vi "ProdaNG.CheckProductExists.vi"(8 "error in (no error)":errorcluster, 9 "serialNumber":string, 10 "ID":T2, 11 "dbHandle":i32) -> (0 "error out":errorcluster, 1 "ProductID":T1, 2 "Results exist?":bool, 3 "dbHandle out":i32, 5 "Prod exist?":bool, 7 "Prod status":i32)   [LabVIEW 2016]
doc: "This function returns a product structure for a product, which is identified by a part and a serial number.\nImportant information: The field 'individual' was taken over from the field 'allgemein' of the legacy data directly. Because of this most products have the value 0 further on and only a few the value 1. \nParameter:\nhandle is an Integer, which is returned by the function Login() at the creation of a new connection.\nwabcoPartId is the Id of the part.\nserialNumber is the serial number of the product for the part above.\nproduct is a pointer on a product structure, which is filled if the returncode is 0. The structure must be defined in the calling program.\n\nReturncodes:\n0 No error\n< 0 ORACLE Error code\n6 (ERROR_INVALID_HANDLE) in case of an invalid handle\n1403 Record does not exist"
uses:
  Controls/ProdaNG.Identification.ctl
  Controls/ProdaNG.Product.ctl
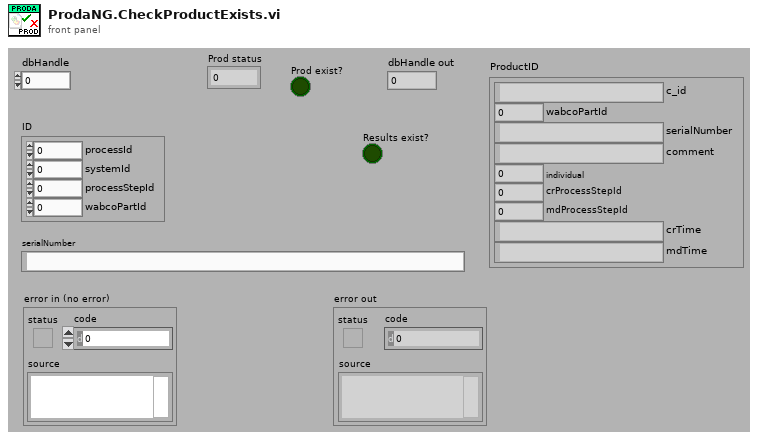
[diagram p1: front panel]
types:
  T1 = typedef "ProdaNG.Product.ctl" = cluster{"c_id":string, "wabcoPartId":i32, "serialNumber":string, "comment":string, "individual":i32, "crProcessStepId":i32, "mdProcessStepId":i32, "crTime":string, "mdTime":string}
  T2 = typedef "ProdaNG.Identification.ctl" = cluster{"processId":i32, "systemId":i32, "processStepId":i32, "wabcoPartId":i32}
  T3 = typedef "ProdaNG.ProcessResult.ctl" = cluster{"c_id":string, "productId":string, "processId":i32, "statusId":i32, "startTime":string, "endTime":string}
  T4 = typedef "ProdaNG.ProcessStepResult.ctl" = cluster{"c_id":string, "processResultId":string, "processStepId":i32, "statusId":i32, "operatorId":i32, "startTime":string, "endTime":string}
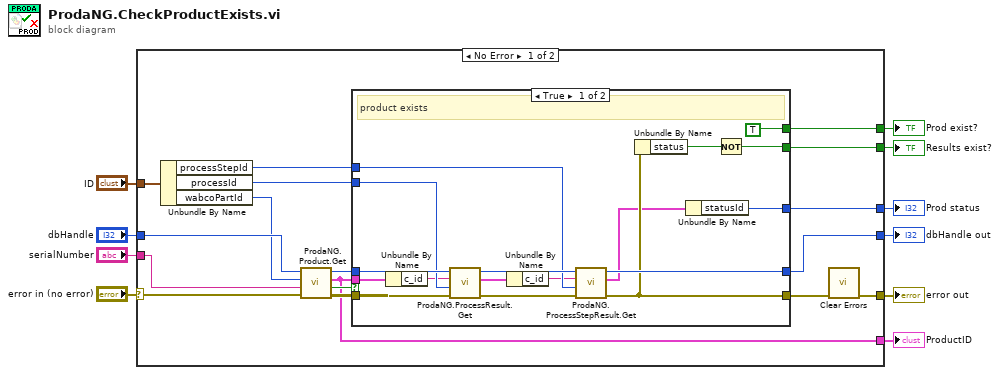
[diagram p0: block diagram]
diagram:
  n1 = case shown="No Error" "error in (no error)" {
    selector: "error in (no error)" -> [w27 w48]
    tunnel: [w15 w48] -> w9
    tunnel: "dbHandle" -> [w24 w47]
    tunnel: [w12 w47] -> w7
    tunnel: "serialNumber" -> [w21 _]
    tunnel: "ID" -> [w23 _]
    tunnel: [w20 _] -> w4
    tunnel: [w14 _] -> w3
    tunnel: [w13 _] -> w2
    tunnel: [w11 _] -> w1
    frame No Error {
      n2 = Unbundle By Name(w23) -> ("processStepId"=w17:i32, "processId"=w18:i32, "wabcoPartId"=w22:i32)
      n3 = call "ProdaNG.Product.Get.vi"("error in (no error)"=w27, "serialNumber"=w21, "wabcoPartId"=w22, "dbHandle"=w24) -> ("error out"=w26:errorcluster, "found"=w25:bool, "Product"=w14:T1, "dbHandle out"=w19:i32)  [unwired: 4 in]
      n4 = case shown="True" w25 {
        tunnel: w26 -> [w39 w46]
        tunnel: [w36 w46] -> w16
        tunnel: [w43 _] -> w20
        tunnel: w19 -> [w38 w45]
        tunnel: [w37 w45] -> w12
        tunnel: w18 -> [w32 _]
        tunnel: w17 -> [w33 _]
        tunnel: w14 -> [w35 _]
        tunnel: [TRUE _] -> w13
        tunnel: [w28 _] -> w11
        frame True {
          # "product exists"
          n5 = Unbundle By Name(w35) -> ("c_id"=w31:string)
          n6 = call "ProdaNG.ProcessResult.Get.vi"("error in (no error)"=w39, "processId"=w32, "productId"=w31, "dbHandle"=w38) -> ("error out"=w40:errorcluster, "ProcessResult"=w42:T3, "dbHandle out"=w41:i32)  [unwired: 4 in, 1 out]
          n7 = Unbundle By Name(w42) -> ("c_id"=w30:string)
          n8 = call "ProdaNG.ProcessStepResult.Get.vi"("error in (no error)"=w40, "processStepId"=w33, "processResultId"=w30, "dbHandle"=w41) -> ("error out"=w36:errorcluster, "ProcessStepResult"=w29:T4, "dbHandle out"=w37:i32)  [unwired: 4 in, 1 out]
          n9 = Unbundle By Name(w36) -> ("status"=w44:bool)
          n10 = Unbundle By Name(w29) -> ("statusId"=w28:i32)
          n11 = Not(x=w44) -> (.not. x?=w43:bool)
        }
        frame False {
          # "product missing"
        }
      }
      n12 = call <vilib>:"Clear Errors.vi"("error in (no error)"=w16) -> ("error out"=w15:errorcluster)  [unwired: 5 in, 1 out]
    }
    frame Error {
    }
  }
  "error out" <- w9
  "dbHandle out" <- w7
  "Results exist?" <- w4
  "ProductID" <- w3
  "Prod exist?" <- w2
  "Prod status" <- w1
